vi "EC_switch_flow_path_subVI_BM.vi"(8 "BoardNum":u32, 11 "Switch Flow Path":bool) -> ()   [LabVIEW 2021]
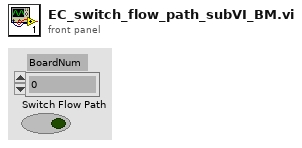
[diagram p1: front panel]
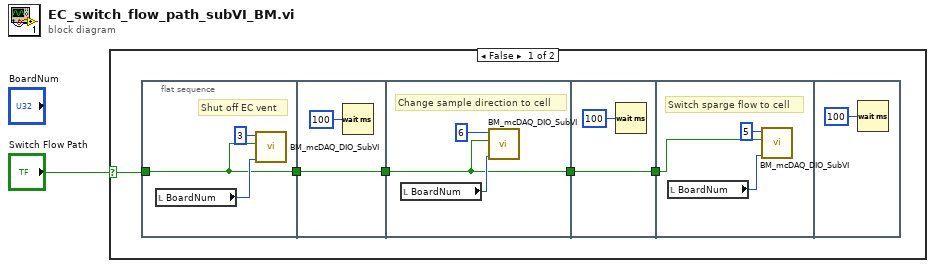
[diagram p0: block diagram]
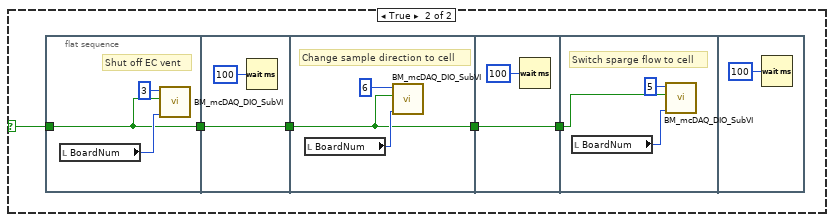
[diagram p2: hidden frame]
diagram:
  n1 = case shown="False" "Switch Flow Path" {
    selector: "Switch Flow Path" -> [w2 w25]
    frame False {
      n2 = flat-sequence {
        tunnel: w2 -> [w7]
        tunnel: [w7] -> w6
        tunnel: w6 -> [w10]
        tunnel: [w10] -> w5
        tunnel: w5 -> [w12]
        tunnel: [w12] -> w4
        tunnel: w4 -> [w15]
        tunnel: [w15] -> w3
        tunnel: w3 -> [w17]
        frame #0 {
          # "Shut off EC vent"
          n3 = local read "BoardNum"() -> (w8:u32)
          n4 = call "BM_mcDAQ_DIO_SubVI.vi"("BoardNum"=w8, "BitValue"=w7, "BitNum"=u32 3) -> ()  [unwired: 8 in, 1 out]
        }
        frame #1 {
          n5 = Wait (ms)(milliseconds to wait=u32 100) -> ()  [unwired: 1 out]
        }
        frame #2 {
          # "Change sample direction to cell"
          n6 = local read "BoardNum"() -> (w13:u32)
          n7 = call "BM_mcDAQ_DIO_SubVI.vi"("BoardNum"=w13, "BitValue"=w12, "BitNum"=u32 6) -> ()  [unwired: 8 in, 1 out]
        }
        frame #3 {
          n8 = Wait (ms)(milliseconds to wait=u32 100) -> ()  [unwired: 1 out]
        }
        frame #4 {
          # "Switch sparge flow to cell"
          n9 = local read "BoardNum"() -> (w18:u32)
          n10 = call "BM_mcDAQ_DIO_SubVI.vi"("BoardNum"=w18, "BitValue"=w17, "BitNum"=u32 5) -> ()  [unwired: 8 in, 1 out]
        }
        frame #5 {
          n11 = Wait (ms)(milliseconds to wait=u32 100) -> ()  [unwired: 1 out]
        }
      }
    }
    frame True {
      n12 = flat-sequence {
        tunnel: w25 -> [w26]
        tunnel: [w26] -> w24
        tunnel: w24 -> [w29]
        tunnel: [w29] -> w23
        tunnel: w23 -> [w31]
        tunnel: [w31] -> w22
        tunnel: w22 -> [w34]
        tunnel: [w34] -> w21
        tunnel: w21 -> [w36]
        frame #0 {
          # "Shut off EC vent"
          n13 = local read "BoardNum"() -> (w27:u32)
          n14 = call "BM_mcDAQ_DIO_SubVI.vi"("BoardNum"=w27, "BitValue"=w26, "BitNum"=u32 3) -> ()  [unwired: 8 in, 1 out]
        }
        frame #1 {
          n15 = Wait (ms)(milliseconds to wait=u32 100) -> ()  [unwired: 1 out]
        }
        frame #2 {
          # "Change sample direction to cell"
          n16 = local read "BoardNum"() -> (w32:u32)
          n17 = call "BM_mcDAQ_DIO_SubVI.vi"("BoardNum"=w32, "BitValue"=w31, "BitNum"=u32 6) -> ()  [unwired: 8 in, 1 out]
        }
        frame #3 {
          n18 = Wait (ms)(milliseconds to wait=u32 100) -> ()  [unwired: 1 out]
        }
        frame #4 {
          # "Switch sparge flow to cell"
          n19 = local read "BoardNum"() -> (w37:u32)
          n20 = call "BM_mcDAQ_DIO_SubVI.vi"("BoardNum"=w37, "BitValue"=w36, "BitNum"=u32 5) -> ()  [unwired: 8 in, 1 out]
        }
        frame #5 {
          n21 = Wait (ms)(milliseconds to wait=u32 100) -> ()  [unwired: 1 out]
        }
      }
    }
  }
